vi "VNA_Get_Trigger.vi"(0 "VISA in":refnum<visa-resource-name>, 1 "error in (no error)":errorcluster) -> (2 "VISA out":refnum<visa-resource-name>, 3 "MODE":string, 4 "error out":errorcluster)   [LabVIEW 2017]
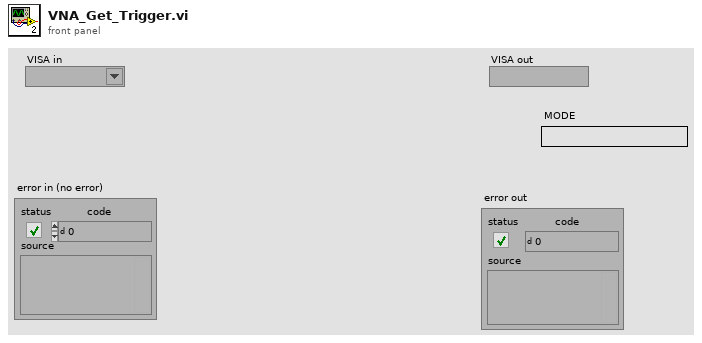
[diagram p1: front panel]
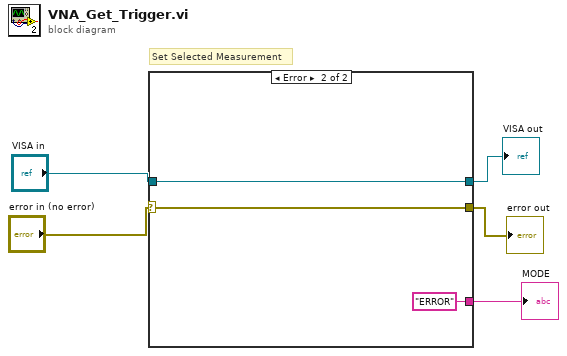
[diagram p0: block diagram]
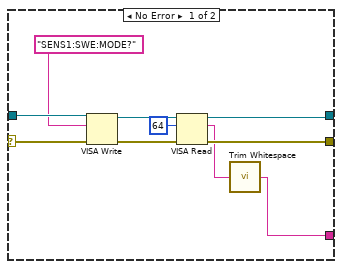
[diagram p2: hidden frame]
diagram:
  # "Set Selected Measurement"
  n1 = case shown="Error" "error in (no error)" {
    selector: "error in (no error)" -> [w15 w18]
    tunnel: [w10 w18] -> w3
    tunnel: "VISA in" -> [w14 w17]
    tunnel: [w11 w17] -> w2
    tunnel: [w6 "ERROR" ("trimmed string")] -> w1
    frame No Error {
      n2 = VISA Write(VISA resource name=w14, write buffer="SENS1:SWE:MODE?" ("Cmdline"), error in (no error)=w15) -> (VISA resource name out=w12:refnum<visa-resource-name>, error out=w9:errorcluster)  [unwired: 1 out]
      n3 = VISA Read(VISA resource name=w12, byte count=u32 64, error in (no error)=w9) -> (VISA resource name out=w11:refnum<visa-resource-name>, read buffer=w7:string, error out=w10:errorcluster)  [unwired: 1 out]
      n4 = call <vilib>:"Trim Whitespace.vi"("string"=w7) -> ("trimmed string"=w6:string)  [unwired: 1 in]
    }
    frame Error {
    }
  }
  "error out" <- w3
  "VISA out" <- w2
  "MODE" <- w1
